vi "Dispatch Tx Transfer Group.vi"(8 "error in (no error)":errorcluster, 9 "Transfer Group ID":i32, 10 "Plugin ID":i32, 11 "Dispatcher Interface in":refnum<class "Dispatcher Interface.lvclass">) -> (0 "error out":errorcluster, 3 "Dispatcher Interface out":refnum<class "Dispatcher Interface.lvclass">)   [LabVIEW 2017, in "DSF Core.lvlib" / "Dispatcher Interface.lvclass"]
uses:
  Interfaces/Dispatcher/Dispatcher Interface.lvclass
  Interfaces/Dispatcher/Tx Parameters.ctl
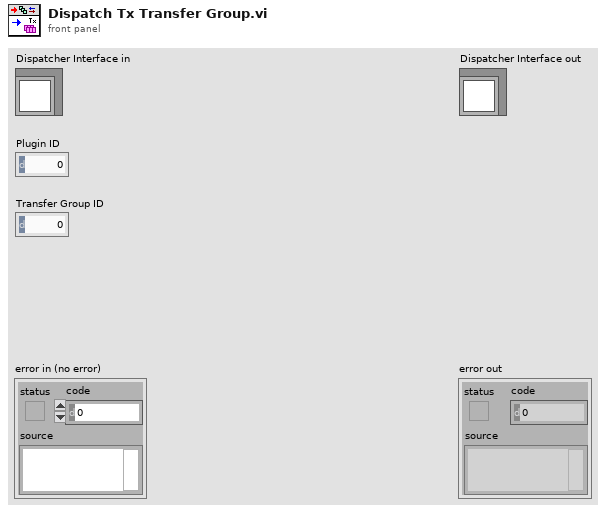
[diagram p1: front panel]
types:
  T1 = typedef "DSF Core.lvlib/Dispatcher Interface.lvclass/Tx Parameters.ctl" = cluster{"Plugin ID":i32, "Transfer Group ID":i32, "Iteration":u64}
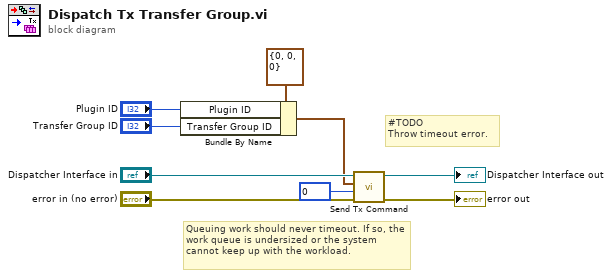
[diagram p0: block diagram]
diagram:
  # "Queuing work should never timeout. If so, the work queue is undersized or the system cannot keep up with the workload."
  # "#TODO\nThrow timeout error."
  n1 = Bundle By Name(cluster=T1 {"Plugin ID"=0, "Transfer Group ID"=0, "Iteration"=0} ("Tx Parameters"), "Plugin ID"="Plugin ID", "Transfer Group ID"="Transfer Group ID") -> (w4:T1)
  n2 = call "Send Tx Command.vi"("error in (no error)"="error in (no error)", "timeout in ms (0)"=0, "Tx Parameters"=w4, "Dispatcher Interface in"="Dispatcher Interface in") -> ("error out"=→"error out":errorcluster, "Dispatcher Interface out"=→"Dispatcher Interface out":refnum<class "Dispatcher Interface.lvclass">)  [unwired: 6 in]
